vi "Secondary System - GamepadPID.vi"() -> ()   [LabVIEW 2011]
uses:
  Team Code/Robot Global Data.vi
  <vilib>/addons/control/pid/pid.llb/PID (DBL).vi
  <vilib>/addons/control/pid/NI_PID_pid.lvlib
panel:
  in  "Arm Constants":T1={"Top Center Peg"=166.0, "Top Outer Pegs"=155.0, "Middle Center Peg"=118.0, "Middle Outer Pegs"=109.0, "Lower Center Peg"=76.0, "Lower Outside Pegs"=73.0, "Feed"=20.0, "Floor"=13.0}
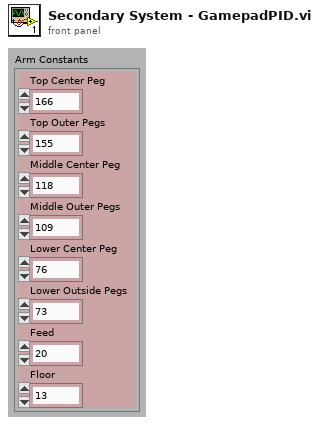
[diagram p1: front panel]
types:
  T1 = cluster{"Top Center Peg":dbl, "Top Outer Pegs":dbl, "Middle Center Peg":dbl, "Middle Outer Pegs":dbl, "Lower Center Peg":dbl, "Lower Outside Pegs":dbl, "Feed":dbl, "Floor":dbl}
  T2 = typedef "Arm Joystick.ctl" = cluster{"Buttons":T3, "Axes":cluster{"axis 1 (x)":dbl, "axis 2 (y)":dbl, "axis 3 (throttle)":dbl, "axis 4":dbl, "axis 5":dbl, "axis 6":dbl}}
  T3 = typedef "WPI_JoystickButtonState.ctl" = cluster{"Button 1":bool, "Button 2":bool, "Button 3":bool, "Button 4":bool, "Button 5":bool, "Button 6":bool, "Button 7":bool, "Button 8":bool, "Button 9":bool, "Button 10":bool, "Button 11":bool, "Button 12":bool}
  T4 = cluster{"proportional gain (Kc)":dbl, "integral time (Ti, min)":dbl, "derivative time (Td, min)":dbl}
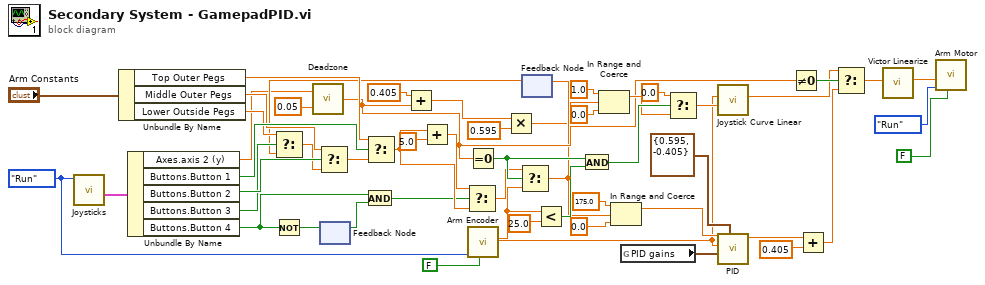
[diagram p0: block diagram]
diagram:
  w53 = enum16{"Init", "Run", "End"}."Run" ("Mode")
  n1 = call "Joysticks.vi"("Mode"=w53) -> ("Arm Joystick"=w51:T2)  [unwired: 8 out]
  n2 = Unbundle By Name("Arm Constants") -> ("Top Outer Pegs"=w34:dbl, "Middle Outer Pegs"=w33:dbl, "Lower Outside Pegs"=w32:dbl)
  n3 = Unbundle By Name(w51) -> ("Axes.axis 2 (y)"=w14:dbl, "Buttons.Button 1"=w40:bool, "Buttons.Button 2"=w39:bool, "Buttons.Button 3"=w38:bool, "Buttons.Button 4"=w17:bool)
  n4 = Not(x=w17) -> (.not. x?=w19:bool)
  n5 = call "Deadzone.vi"("Deadzone"=0.05, "Input"=w14) -> ("Output"=w13:dbl)
  n6 = feedback-in #1(w19) -> ()
  n7 = feedback #1() -> (w18:bool)  [unwired: 1 out]
  n8 = And(x=w17, y=w18) -> (x .and. y?=w16:bool)
  n9 = Add(x=0.405 ("y"), y=w13) -> (x+y=w4:dbl)
  n10 = Equal To 0?(x=w13) -> (x = 0?=w28:bool)
  n11 = call "Arm Encoder.vi"("Reset Encoder?"=FALSE, "Mode"=w53) -> ("Get Arm Encoder"=w2:dbl)  [unwired: 1 in, 8 out]
  n12 = Multiply(x=w4, y=0.595) -> (x*y=w5:dbl)
  n13 = feedback #2() -> (w26:dbl)  [unwired: 1 out]
  n14 = Select(t=w32, s=w38, f=w26) -> (s? t:f=w36:dbl)
  n15 = Select(t=w33, s=w39, f=w36) -> (s? t:f=w37:dbl)
  n16 = Select(t=w34, s=w40, f=w37) -> (s? t:f=w29:dbl)
  n17 = Add(x=w29, y=5.0) -> (x+y=w31:dbl)
  n18 = Select(t=w31, s=w16, f=w29) -> (s? t:f=w27:dbl)
  n19 = Select(t=w27, s=w28, f=w2) -> (s? t:f=w9:dbl)
  n20 = feedback-in #2(w9) -> ()
  n21 = Less?(x=w2, y=25.0) -> (x < y?=w46:bool)
  n22 = And(x=w28, y=w46) -> (x .and. y?=w45:bool)
  n23 = In Range and Coerce(upper limit=1.0, x=w5, lower limit=0.0) -> (coerced(x)=w43:dbl)  [unwired: 1 out]
  n24 = In Range and Coerce(upper limit=175.0, x=w9, lower limit=0.0) -> (coerced(x)=w8:dbl)  [unwired: 1 out]
  n25 = global read "Robot Global Data.vi" "PID gains"() -> (w20:T4)
  n26 = Select(t=0.0, s=w45, f=w43) -> (s? t:f=w3:dbl)
  n27 = call "Joystick Curve Linear.vi"("Joystick Input"=w3, "Encoder Input"=w2) -> ("Motor Output"=w1:dbl)  [unwired: 9 out]
  n28 = call-poly <vilib>:"PID.vi"("output range"=cluster{"output high":dbl, "output low":dbl} {"output high"=0.595, "output low"=-0.405}, "PID gains"=w20, "process variable"=w2, "setpoint"=w8) -> ("output"=w23:dbl)  [unwired: 2 in, 5 out]
  n29 = Not Equal To 0?(x=w13) -> (x != 0?=w24:bool)
  n30 = Add(x=w23, y=0.405) -> (x+y=w21:dbl)
  n31 = Select(t=w1, s=w24, f=w21) -> (s? t:f=w12:dbl)
  n32 = call "Victor Linearize.vi"("Goal Speed"=w12) -> ("Output"=w11:dbl)  [unwired: 10 out]
  n33 = call "Arm Motor.vi"("Stall Arm?"=FALSE, "Mode"=enum16{"Init", "Run", "End"}."Run", "Arm motor speed"=w11) -> ()  [unwired: 1 in, 8 out]
